vi "Buffer Manager.vi"(6 "Number of Samples":i32=50000, 7 "Function":T1, 8 "error in":errorcluster, 9 "Unique Channel Identifier":string, 10 "Waveform in":waveform(dbl), 11 "Plugin in":refnum<class "Power Spectrum Density.lvclass">) -> (0 "error out":errorcluster, 1 "Data Valid":bool, 2 "Waveform out":waveform(dbl), 3 "Plugin out":refnum<class "Power Spectrum Density.lvclass">, 4 "Percentage":dbl)   [LabVIEW 2023, in "Power Spectrum Density.lvlib" / "Power Spectrum Density.lvclass"]
uses:
  Power Spectrum Density.lvclass
  Buffer Manager Function.ctl
  C:/Program Files/National Instruments/LabVIEW 2023/vi.lib/FlexLogger/SDK/PluginSDK.lvlibp/PEFClasses/SDK/Processing Element/Processing Element.lvclass
  <vilib>/FlexLogger/SDK/PluginSDK.lvlibp/PEFClasses/SDK/Processing Element/Read Alias.vi
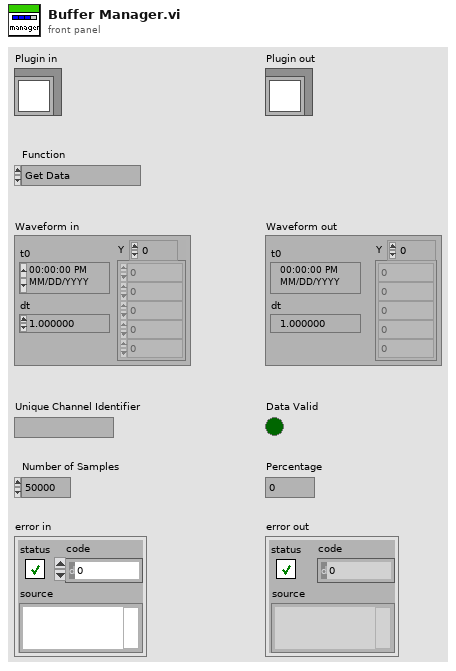
[diagram p1: front panel]
types:
  T1 = typedef "Power Spectrum Density.lvlib/Power Spectrum Density.lvclass/Buffer Manager Function.ctl" = enum16{"Get Data", "Buffer Data", "Reset Data"}
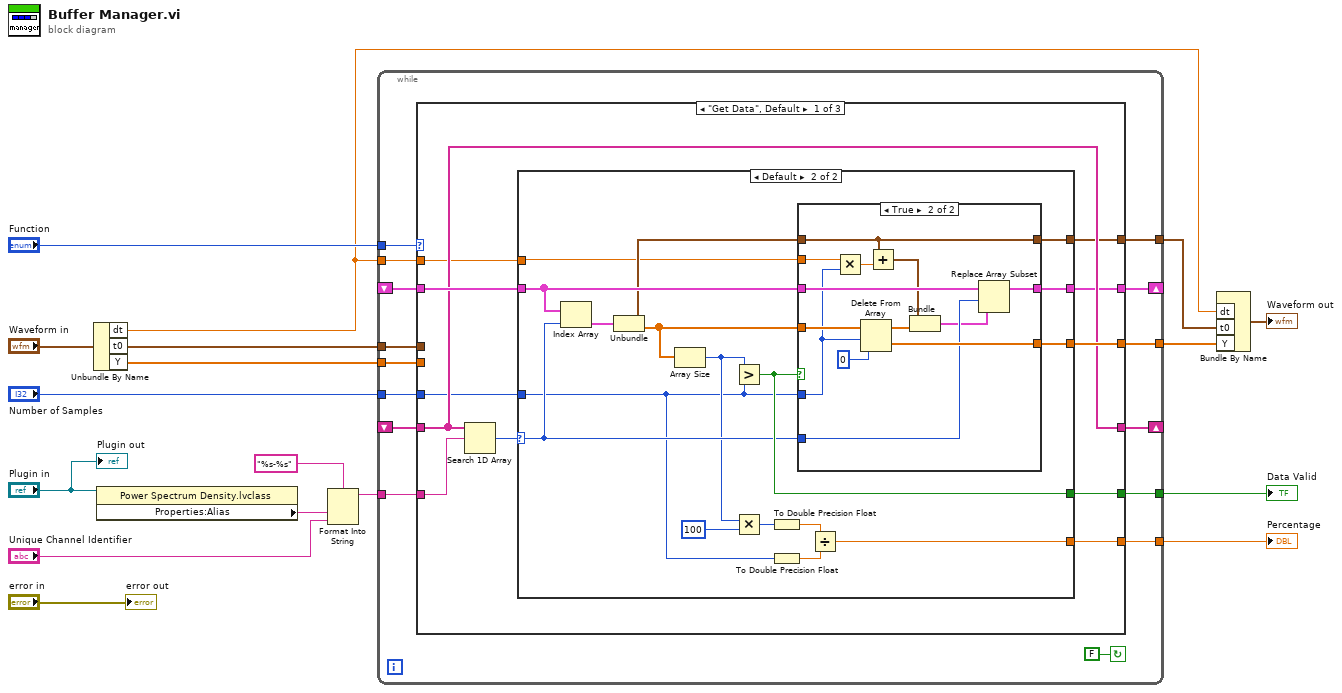
[diagram p0: block diagram]
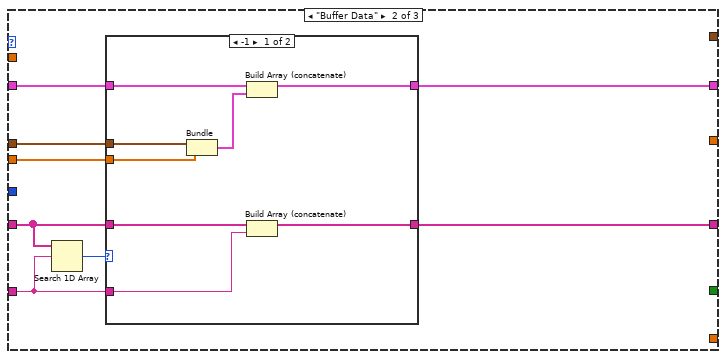
[diagram p4: hidden frame]
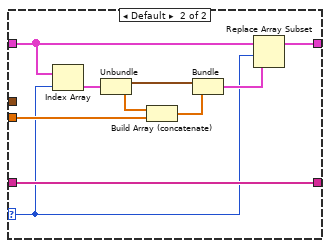
[diagram p5: hidden frame]
diagram:
  n1 = Unbundle By Name("Waveform in") -> ("dt"=w2:dbl, "t0"=w4:timestamp, "Y"=w10:dbl[])
  n2 = property class="Power Spectrum Density.lvclass"(reference="Plugin in") -> ("Properties:Alias"=w14:string)  [unwired: 1 in, 2 out]
  n3 = Format Into String(format string="%s-%s", w14, "Unique Channel Identifier") -> (resulting string=w13:string)  [unwired: 2 in, 1 out]
  n4 = while {
    tunnel: "Function" -> [w32]
    shift-right: [w25] -> _
    shift-left: _ -> [w31]
    shift-right: [w24] -> _
    shift-left: _ -> [w28]
    tunnel: w13 -> [w30]
    tunnel: [w29] -> w11
    tunnel: [w27] -> w6
    tunnel: w10 -> [w26]
    tunnel: "Number of Samples" -> [w22]
    tunnel: w4 -> [w21]
    tunnel: [w20] -> w3
    tunnel: w2 -> [w19]
    tunnel: [w18] -> w1
    stop <- FALSE continue-if-true
    n5 = case shown="\"Get Data\", Default" w32 {
      tunnel: w31 -> [w38 w81 _]
      tunnel: w30 -> [w43 w80 _]
      tunnel: [w41 _ _] -> w29
      tunnel: w28 -> [w39 w82 _]
      tunnel: [w40 _ _] -> w27
      tunnel: w26 -> [_ w77 _]
      tunnel: [w38 w79 _] -> w25
      tunnel: [w37 w78 _] -> w24
      tunnel: w22 -> [w36 _ _]
      tunnel: w21 -> [_ w76 _]
      tunnel: [w35 _ _] -> w20
      tunnel: w19 -> [w34 _ _]
      tunnel: [w33 _ _] -> w18
      frame "Get Data", Default {
        n6 = Search 1D Array(1D array=w38, element=w43) -> (index of element=w42:i32)  [unwired: 1 in]
        n7 = case shown="Default" w42 {
          selector: w42 -> [_ w58]
          tunnel: [_ w60] -> w41
          tunnel: w39 -> [w44 w57]
          tunnel: w36 -> [_ w48]
          tunnel: [_ w59] -> w40
          tunnel: [w44 w56] -> w37
          tunnel: [_ w54] -> w35
          tunnel: w34 -> [_ w52]
          tunnel: [_ w45] -> w33
          frame -1 {
          }
          frame Default {
            n8 = Index Array(array=w57, index=w58) -> (element=w61:cluster{"t0":timestamp, "Y":dbl[]})
            n9 = Unbundle(w61) -> ("t0"=w53:timestamp, "Y"=w55:dbl[])
            n10 = Array Size(array=w55) -> (size(s)=w51:i32)
            n11 = Greater?(x=w51, y=w48) -> (0:w60:bool)
            n12 = Multiply(x=w51, y=100) -> (x*y=w49:i32)
            n13 = To Double Precision Float(number=w49) -> (double precision float=w47:dbl)
            n14 = To Double Precision Float(number=w48) -> (double precision float=w46:dbl)
            n15 = case shown="True" w60 {
              tunnel: w55 -> [_ w74]
              tunnel: w48 -> [_ w66]
              tunnel: [_ w75] -> w59
              tunnel: w58 -> [_ w71]
              tunnel: w57 -> [w62 w70]
              tunnel: [w62 w68] -> w56
              tunnel: [_ w67] -> w54
              tunnel: w53 -> [_ w67]
              tunnel: w52 -> [_ w65]
              frame False {
              }
              frame True {
                n16 = Multiply(x=w65, y=w66) -> (x*y=w64:dbl)
                n17 = Delete From Array(array=w74, length=w66, index=0) -> (deleted portion=w75:dbl[], array with subset deleted=w72:dbl[])
                n18 = Add(x=w67, y=w64) -> (x+y=w63:timestamp)
                n19 = Bundle(w63, "Y"=w72) -> (w69:cluster{timestamp, "Y":dbl[]})  [unwired: 1 in]
                n20 = Replace Array Subset(array=w70, new element=w69, index=w71) -> (w68:cluster{"t0":timestamp, "Y":dbl[]}[])
              }
            }
            n21 = Divide(x=w47, y=w46) -> (x/y=w45:dbl)
          }
        }
      }
      frame "Buffer Data" {
        n22 = Search 1D Array(1D array=w81, element=w80) -> (index of element=w83:i32)  [unwired: 1 in]
        n23 = case shown="-1" w83 {
          selector: w83 -> [_ w94]
          tunnel: w82 -> [w88 w98]
          tunnel: w81 -> [w91 w95]
          tunnel: w80 -> [w90 _]
          tunnel: [w89 w95] -> w79
          tunnel: [w87 w96] -> w78
          tunnel: w77 -> [w86 w100]
          tunnel: w76 -> [w84 _]
          frame -1 {
            n24 = Bundle("t0"=w84, "Y"=w86) -> (w85:cluster{"t0":timestamp, "Y":dbl[]})  [unwired: 1 in]
            n25 = Build Array (concatenate)(w88, w85) -> (w87:cluster{"t0":timestamp, "Y":dbl[]}[])
            n26 = Build Array (concatenate)(w91, w90) -> (w89:string[])
          }
          frame Default {
            n27 = Index Array(array=w98, index=w94) -> (element=w101:cluster{"t0":timestamp, "Y":dbl[]})
            n28 = Unbundle(w101) -> ("t0"=w92:timestamp, "Y"=w93:dbl[])
            n29 = Build Array (concatenate)(w93, w100) -> (w99:dbl[])
            n30 = Bundle("t0"=w92, w99) -> (w97:cluster{"t0":timestamp, dbl[]})  [unwired: 1 in]
            n31 = Replace Array Subset(array=w98, new element=w97, index=w94) -> (w96:cluster{"t0":timestamp, "Y":dbl[]}[])
          }
        }
      }
      frame "Reset Data" {
      }
    }
  }
  "Data Valid" <- w11
  "Percentage" <- w1
  n32 = Bundle By Name("dt"=w2, "t0"=w3, "Y"=w6) -> (→"Waveform out":waveform(dbl))  [unwired: 1 in]
  "error out" <- "error in"
  "Plugin out" <- "Plugin in"
